vi "DigitalClock.vi"() -> ()   [LabVIEW 2018]
panel:
  in  "stop":bool
  out "A":bool caption="Boolean"
  out "F":bool caption="Boolean 2"
  out "G":bool caption="Boolean 3"
  out "Boolean 4":bool
  out "B":bool caption="Boolean 6"
  out "C":bool caption="Boolean 7"
  out "D":bool caption="Boolean 8"
  out "Boolean 32":bool
  out "Boolean 31":bool
  out "Boolean 30":bool
  out "Boolean 29":bool
  out "Boolean 28":bool
  out "Boolean 27":bool
  out "Boolean 26":bool
  out "Boolean 24":bool
  out "Boolean 23":bool
  out "Boolean 22":bool
  out "Boolean 21":bool
  out "Boolean 20":bool
  out "Boolean 19":bool
  out "Boolean 18":bool
  out "Boolean 16":bool
  out "Boolean 15":bool
  out "Boolean 14":bool
  out "Boolean 13":bool
  out "Boolean 12":bool
  out "Boolean 11":bool
  out "Boolean 10":bool
  out "Boolean 34":bool
  out "Boolean 33":bool
  out "A-L":bool caption="Boolean 16"
  out "F-L":bool caption="Boolean 15"
  out "G-L":bool caption="Boolean 14"
  out "E-L":bool caption="Boolean 13"
  out "B-L":bool caption="Boolean 12"
  out "C-L":bool caption="Boolean 11"
  out "D-L":bool caption="Boolean 10"
  out "A-M":bool caption="Boolean 16"
  out "F-M":bool caption="Boolean 15"
  out "G-M":bool caption="Boolean 14"
  out "E-M":bool caption="Boolean 13"
  out "B-M":bool caption="Boolean 12"
  out "C-M":bool caption="Boolean 11"
  out "D-M":bool caption="Boolean 10"
  out "Boolean 52":bool
  out "Boolean 51":bool
  out "DP":bool
  out "Boolean 25":bool
  out "Boolean 17":bool
  out "Boolean 9":bool
  out "DP-L":bool caption="Boolean 35"
  out "DP-M":bool caption="Boolean 43"
  in  "Delay Time (s)":dbl=1.0
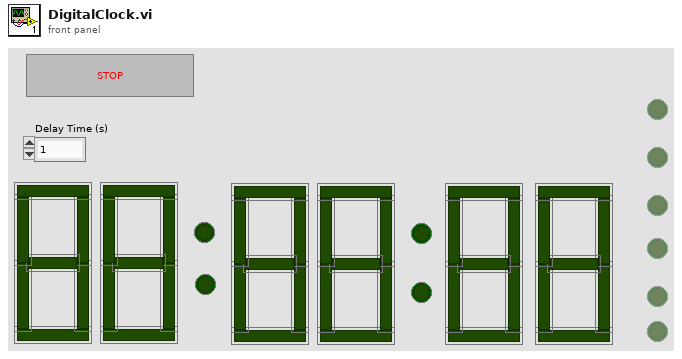
[diagram p1: front panel]
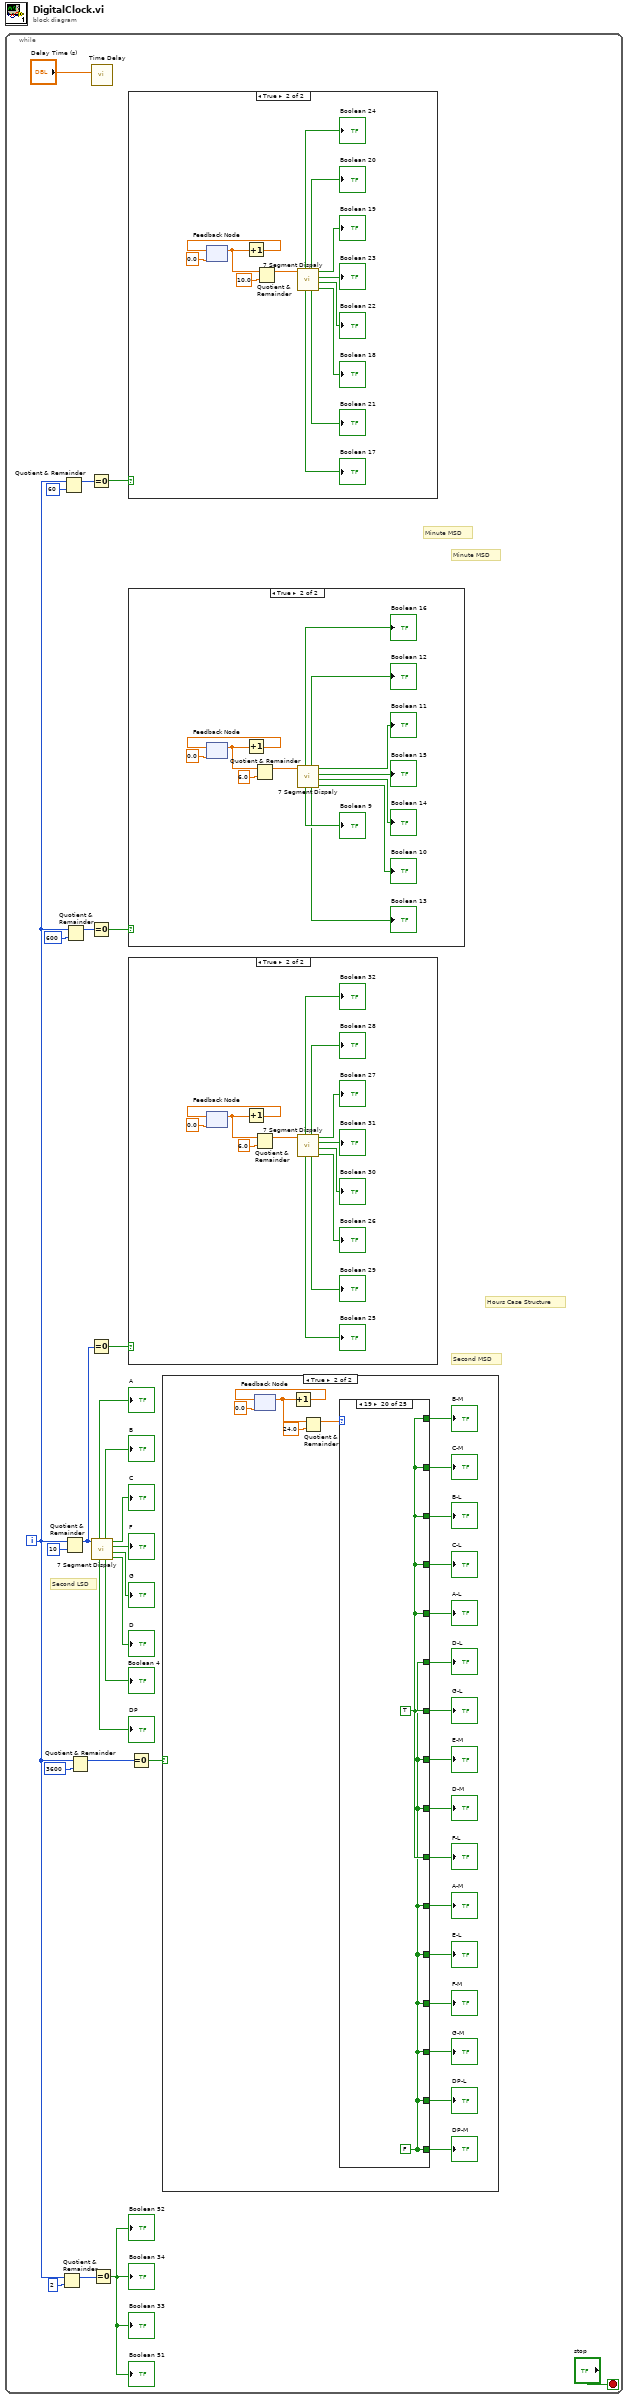
[diagram p0: block diagram]
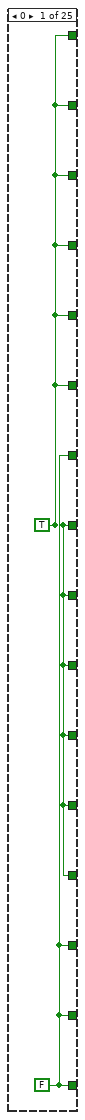
[diagram p3: hidden frame]
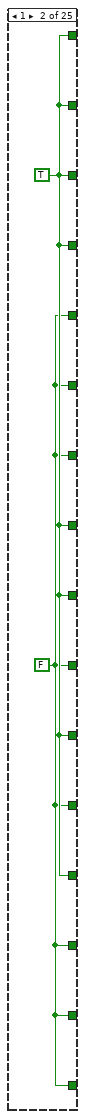
[diagram p4: hidden frame]
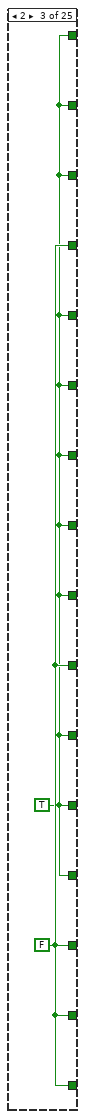
[diagram p5: hidden frame]
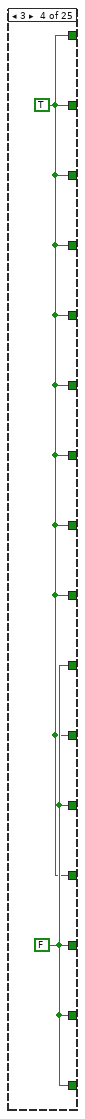
[diagram p6: hidden frame]
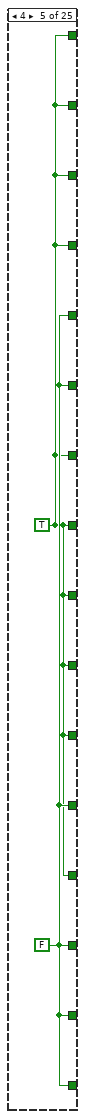
[diagram p7: hidden frame]
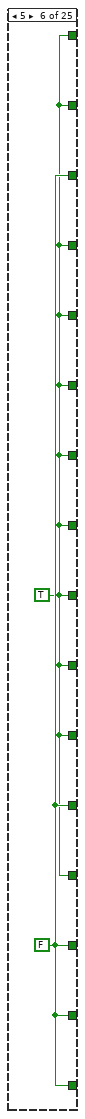
[diagram p8: hidden frame]
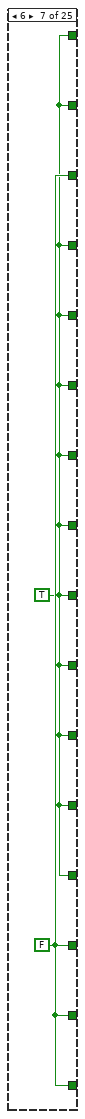
[diagram p9: hidden frame]
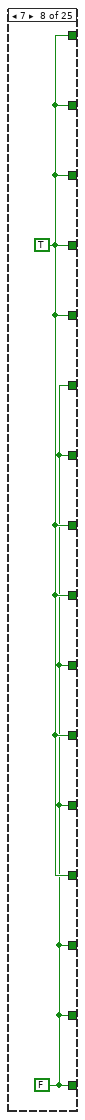
[diagram p10: hidden frame]
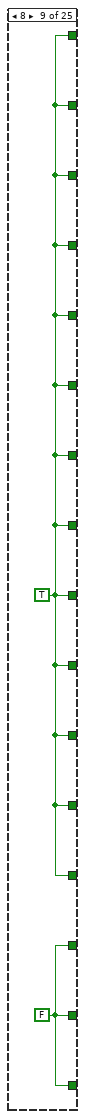
[diagram p11: hidden frame]
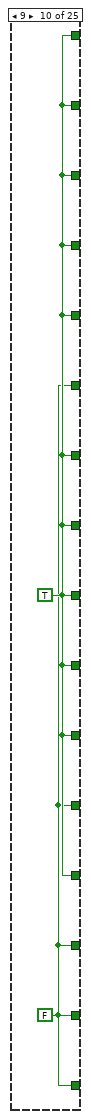
[diagram p12: hidden frame]
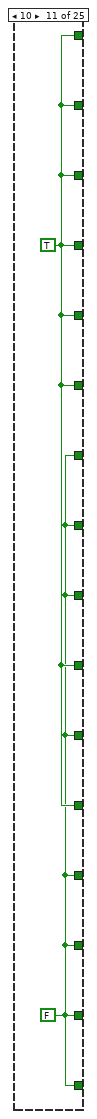
[diagram p13: hidden frame]
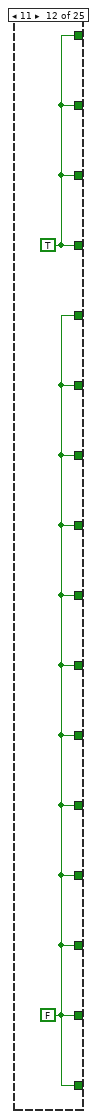
[diagram p14: hidden frame]
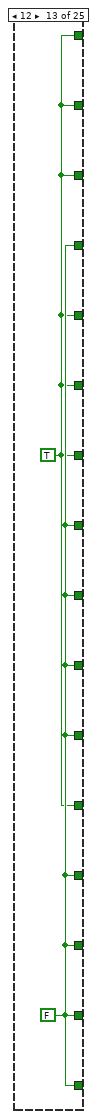
[diagram p15: hidden frame]
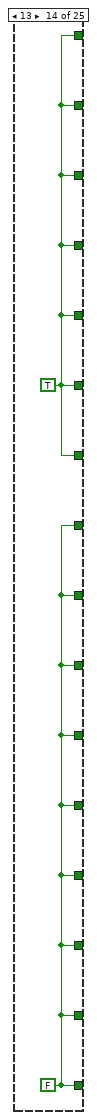
[diagram p16: hidden frame]
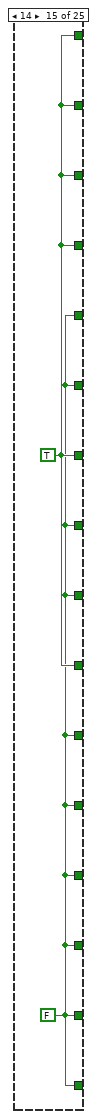
[diagram p17: hidden frame]
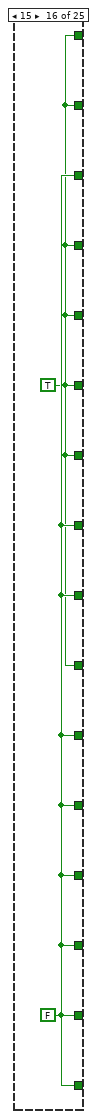
[diagram p18: hidden frame]
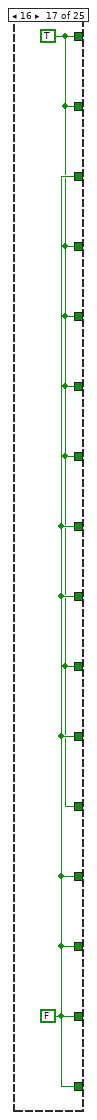
[diagram p19: hidden frame]
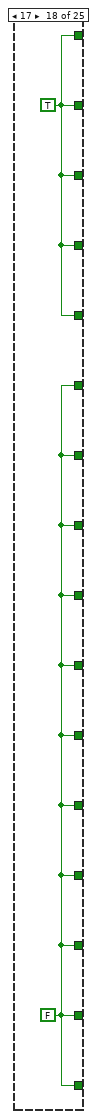
[diagram p20: hidden frame]
diagram:
  n1 = while {
    i -> [w3]
    stop <- "stop" stop-if-true
    # "Minute MSD"
    # "Second MSD"
    # "Second LSD"
    # "Minute MSD"
    # "Hours Case Structure"
    n2 = Quotient & Remainder(x=w3, y=2) -> (x-y*floor(x/y)=w4:i32)  [unwired: 1 out]
    n3 = Quotient & Remainder(x=w3, y=60) -> (x-y*floor(x/y)=w11:i32)  [unwired: 1 out]
    n4 = Quotient & Remainder(x=w3, y=10) -> (x-y*floor(x/y)=w15:i32)  [unwired: 1 out]
    n5 = Quotient & Remainder(x=w3, y=600) -> (x-y*floor(x/y)=w12:i32)  [unwired: 1 out]
    n6 = Quotient & Remainder(x=w3, y=3600 ("N")) -> (x-y*floor(x/y)=w13:i32)  [unwired: 1 out]
    n7 = Equal To 0?(x=w11) -> (x = 0?=w10:bool)
    n8 = Equal To 0?(x=w12) -> (x = 0?=w9:bool)
    n9 = Equal To 0?(x=w15) -> (x = 0?=w16:bool)
    n10 = call "Time Delay"("Delay Time (s)"="Delay Time (s)") -> ()  [unwired: 10 in, 1 out]
    n11 = call "7 Segment Dispaly.vi"("Ring"=w15) -> ("D"=→"D":bool, "G"=→"G":bool, "F"=→"F":bool, "C"=→"C":bool, "E"=→"Boolean 4":bool, "B"=→"B":bool, "DP"=→"DP":bool, "A"=→"A":bool)  [unwired: 3 in]
    n12 = Equal To 0?(x=w4) -> (x = 0?=→"Boolean 34" →"Boolean 33" →"Boolean 52" →"Boolean 51":bool)
    n13 = case shown="True" w10 {
      frame False {
      }
      frame True {
        n14 = feedback #1(0.0) -> (w112:dbl)
        n15 = Increment(x=w112) -> (x+1=w113:dbl)
        n16 = feedback-in #1(w113) -> ()
        n17 = Quotient & Remainder(x=w112, y=10.0) -> (x-y*floor(x/y)=w111:dbl)  [unwired: 1 out]
        n18 = call "7 Segment Dispaly.vi"("Ring"=w111) -> ("D"=→"Boolean 18":bool, "G"=→"Boolean 22":bool, "F"=→"Boolean 23":bool, "C"=→"Boolean 19":bool, "E"=→"Boolean 21":bool, "B"=→"Boolean 20":bool, "DP"=→"Boolean 17":bool, "A"=→"Boolean 24":bool)  [unwired: 3 in]
      }
    }
    n19 = case shown="True" w9 {
      frame False {
      }
      frame True {
        n20 = feedback #2(0.0) -> (w99:dbl)
        n21 = Increment(x=w99) -> (x+1=w100:dbl)
        n22 = feedback-in #2(w100) -> ()
        n23 = Quotient & Remainder(x=w99, y=6.0) -> (x-y*floor(x/y)=w98:dbl)  [unwired: 1 out]
        n24 = call "7 Segment Dispaly.vi"("Ring"=w98) -> ("D"=→"Boolean 10":bool, "G"=→"Boolean 14":bool, "F"=→"Boolean 15":bool, "C"=→"Boolean 11":bool, "E"=→"Boolean 13":bool, "B"=→"Boolean 12":bool, "DP"=→"Boolean 9":bool, "A"=→"Boolean 16":bool)  [unwired: 3 in]
      }
    }
    n25 = case shown="True" w16 {
      frame False {
      }
      frame True {
        n26 = feedback #3(0.0) -> (w128:dbl)
        n27 = Increment(x=w128) -> (x+1=w127:dbl)
        n28 = feedback-in #3(w127) -> ()
        n29 = Quotient & Remainder(x=w128, y=6.0) -> (x-y*floor(x/y)=w125:dbl)  [unwired: 1 out]
        n30 = call "7 Segment Dispaly.vi"("Ring"=w125) -> ("D"=→"Boolean 26":bool, "G"=→"Boolean 30":bool, "F"=→"Boolean 31":bool, "C"=→"Boolean 27":bool, "E"=→"Boolean 29":bool, "B"=→"Boolean 28":bool, "DP"=→"Boolean 25":bool, "A"=→"Boolean 32":bool)  [unwired: 3 in]
      }
    }
    n31 = Equal To 0?(x=w13) -> (x = 0?=w5:bool)
    n32 = case shown="True" w5 {
      frame False {
      }
      frame True {
        n33 = feedback #4(0.0) -> (w47:dbl)
        n34 = Increment(x=w47) -> (x+1=w46:dbl)
        n35 = feedback-in #4(w46) -> ()
        n36 = Quotient & Remainder(x=w47, y=24.0) -> (x-y*floor(x/y)=w43:dbl)  [unwired: 1 out]
        n37 = case shown="19" w43 {
          tunnel: [w49 w50 w53 w55 w57 w59 w61 w62 w65 w66 w68 w71 w73 w74 w76 w79 w81 w82 w85 w86 w89 w91 w92 w95 w96] -> w42
          tunnel: [w49 w50 w53 w55 w57 w59 w61 w62 w65 w66 w68 w71 w73 w74 w76 w79 w81 w82 w85 w86 w89 w91 w92 w95 w96] -> w41
          tunnel: [w48 w51 w52 w54 w56 w58 w60 w63 w64 w67 w68 w71 w73 w74 w76 w79 w81 w82 w85 w86 w88 w90 w93 w94 w97] -> w40
          tunnel: [w48 w51 w52 w54 w56 w58 w60 w63 w64 w67 w68 w71 w73 w74 w76 w79 w81 w82 w85 w86 w88 w90 w93 w94 w97] -> w39
          tunnel: [w49 w50 w53 w55 w57 w59 w61 w62 w65 w66 w68 w71 w73 w74 w76 w79 w81 w82 w85 w86 w88 w90 w93 w94 w97] -> w38
          tunnel: [w48 w51 w52 w54 w56 w58 w60 w63 w64 w67 w69 w70 w72 w75 w77 w78 w80 w83 w84 w87 w89 w91 w92 w95 w97] -> w37
          tunnel: [w48 w51 w52 w54 w56 w58 w60 w63 w64 w67 w68 w71 w73 w74 w76 w79 w81 w82 w85 w86 w89 w91 w92 w95 w97] -> w36
          tunnel: [w48 w51 w52 w54 w56 w58 w60 w63 w64 w67 w69 w70 w72 w75 w77 w78 w80 w83 w84 w87 w88 w90 w93 w94 w97] -> w35
          tunnel: [w48 w51 w52 w54 w56 w58 w60 w63 w64 w67 w68 w71 w73 w74 w76 w79 w81 w82 w85 w86 w88 w90 w93 w94 w97] -> w34
          tunnel: [w49 w50 w52 w54 w56 w58 w60 w62 w64 w67 w68 w71 w72 w75 w77 w78 w80 w82 w84 w87 w89 w91 w93 w94 w97] -> w33
          tunnel: [w48 w50 w52 w54 w57 w58 w60 w62 w64 w66 w69 w71 w72 w75 w76 w78 w80 w82 w84 w86 w88 w91 w93 w94 w97] -> w32
          tunnel: [w48 w50 w52 w55 w57 w59 w60 w62 w64 w66 w69 w71 w72 w74 w76 w79 w80 w82 w84 w86 w88 w91 w93 w95 w97] -> w31
          tunnel: [w48 w51 w53 w54 w56 w58 w60 w63 w64 w67 w69 w70 w73 w75 w77 w78 w80 w83 w84 w87 w88 w90 w92 w94 w97] -> w30
          tunnel: [w48 w50 w53 w55 w56 w58 w60 w62 w64 w67 w69 w71 w73 w74 w77 w78 w80 w82 w84 w87 w88 w91 w92 w95 w97] -> w29
          tunnel: [w48 w51 w52 w54 w56 w59 w61 w63 w64 w67 w69 w70 w72 w75 w77 w79 w81 w83 w84 w87 w88 w90 w93 w94 w97] -> w28
          tunnel: [w48 w50 w52 w54 w57 w58 w60 w63 w64 w67 w69 w71 w72 w75 w76 w78 w80 w83 w84 w87 w88 w91 w93 w94 w97] -> w27
          frame 0 {
            w49 = FALSE
            w48 = TRUE
          }
          frame 1 {
            w50 = FALSE
            w51 = TRUE
          }
          frame 2 {
            w53 = FALSE
            w52 = TRUE
          }
          frame 3 {
            w55 = FALSE
            w54 = TRUE
          }
          frame 4 {
            w57 = FALSE
            w56 = TRUE
          }
          frame 5 {
            w59 = FALSE
            w58 = TRUE
          }
          frame 6 {
            w61 = FALSE
            w60 = TRUE
          }
          frame 7 {
            w62 = FALSE
            w63 = TRUE
          }
          frame 8 {
            w65 = FALSE
            w64 = TRUE
          }
          frame 9 {
            w66 = FALSE
            w67 = TRUE
          }
          frame 10 {
            w68 = FALSE
            w69 = TRUE
          }
          frame 11 {
            w70 = TRUE
            w71 = FALSE
          }
          frame 12 {
            w72 = TRUE
            w73 = FALSE
          }
          frame 13 {
            w74 = FALSE
            w75 = TRUE
          }
          frame 14 {
            w77 = TRUE
            w76 = FALSE
          }
          frame 15 {
            w78 = TRUE
            w79 = FALSE
          }
          frame 16 {
            w80 = TRUE
            w81 = FALSE
          }
          frame 17 {
            w83 = TRUE
            w82 = FALSE
          }
          frame 18 {
            w84 = TRUE
            w85 = FALSE
          }
          frame 19 {
            w87 = TRUE
            w86 = FALSE
          }
          frame 20 {
            w89 = FALSE
            w88 = TRUE
          }
          frame 21 {
            w90 = TRUE
            w91 = FALSE
          }
          frame 22 {
            w92 = FALSE
            w93 = TRUE
          }
          frame 23 {
            w95 = FALSE
            w94 = TRUE
          }
          frame Default {
            w97 = FALSE
            w96 = TRUE
          }
        }
        "A-L" <- w27
        "F-L" <- w29
        "G-L" <- w33
        "E-L" <- w31
        "B-L" <- w28
        "C-L" <- w30
        "D-L" <- w32
        "DP-L" <- w41
        "A-M" <- w34
        "F-M" <- w36
        "G-M" <- w38
        "E-M" <- w40
        "B-M" <- w35
        "C-M" <- w37
        "D-M" <- w39
        "DP-M" <- w42
      }
    }
  }
